vi "Serial.vi"(8 "error in (no error)":errorcluster, 9 "Clear Log":bool, 10 "write buffer":string="UA[3]\r\n", 11 "VISA resource name":refnum<visa-resource-name>="COM6") -> (0 "error out":errorcluster, 2 "read buffer":string, 3 "status":bool)   [LabVIEW 2017]
uses:
  <vilib>/Instr/_visa.llb/VISA Configure Serial Port (Instr).vi
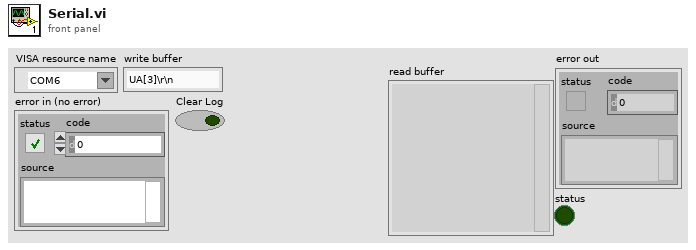
[diagram p1: front panel]
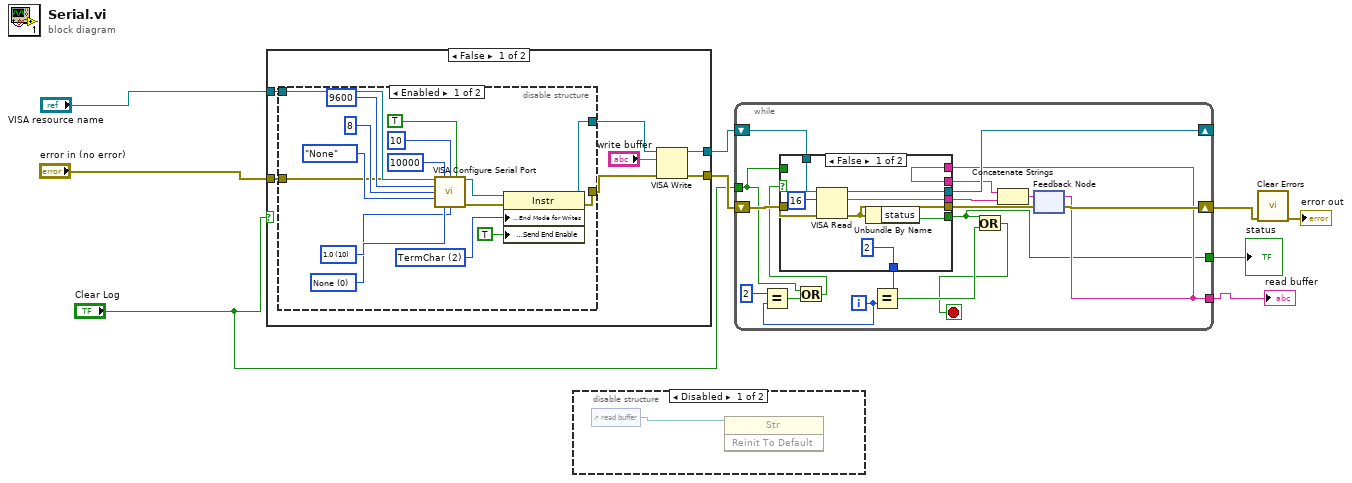
[diagram p0: block diagram]
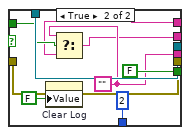
[diagram p5: hidden frame]
diagram:
  n1 = case shown="False" "Clear Log" {
    tunnel: "VISA resource name" -> [w16 w36]
    tunnel: "error in (no error)" -> [w15 w35]
    tunnel: [w12 w36] -> w4
    tunnel: [w11 w35] -> w3
    frame False {
      n2 = disable-structure shown="Enabled" {
        disable-tunnel: w16 -> [w32 w34]
        disable-tunnel: w15 -> [w26 w33]
        disable-tunnel: [w21 w34] -> w13
        disable-tunnel: [w20 w33] -> w14
        frame Enabled {
          w18 = u16 2 items=["None", "LastBit", "TermChar", "Break"] ("Serial Settings:Serial End Mode for Writes")
          w24 = u16 0 items=["None", "XON/XOFF", "RTS/CTS", "XON/XOFF & RTS/CTS", "DTR/DSR", "XON/XOFF & DTR/DSR"] ("flow control (0:none)")
          w25 = u16 10 items=["1.0"=10, "1.5"=15, "2.0"=20] ("stop bits (10: 1 bit)")
          n3 = call-poly "VISA Configure Serial Port"("VISA resource name"=w32, "timeout (10sec)"=u32 10000, "termination char\n(0xA = '\\n' = LF)"=u8 10 ("termination char\n(0xA = '\\n' = LF)"), "Enable Termination\nChar (T)"=TRUE ("Enable Termination\nChar (T)"), "baud rate (9600)"=u32 9600, "data bits (8)"=u16 8, "parity (0:none)"=enum16{"None", "Odd", "Even", "Mark", "Space"}."None", "error in (no error)"=w26, "stop bits (10: 1 bit)"=w25, "flow control (0:none)"=w24) -> ("VISA resource name out"=w22:refnum<visa-resource-name>, "error out"=w23:errorcluster)  [unwired: 4 in]
          n4 = property class="Instr"(reference=w22, error in=w23, "Serial Settings:End Mode for Writes"=w18, "Message Based Settings:Send End Enable"=TRUE) -> (reference out=w21:refnum<visa-resource-name>, error out=w20:errorcluster)
        }
        frame Disabled {
        }
      }
      n5 = VISA Write(VISA resource name=w13, write buffer="write buffer", error in (no error)=w14) -> (VISA resource name out=w12:refnum<visa-resource-name>, error out=w11:errorcluster)  [unwired: 1 out]
    }
    frame True {
    }
  }
  n6 = disable-structure shown="Disabled" {
    frame Disabled {
      n7 = control-ref of="read buffer"() -> (w37:refnum<vi>)
      n8 = invoke class="Str" method="Reinit To Default"(reference=w37) -> ()  [unwired: 2 in, 3 out]
    }
    frame Enabled {
    }
  }
  n9 = while {
    shift-right: [w54] -> _
    shift-left: w4 -> [w49]
    shift-right: [w52] -> w8
    shift-left: w3 -> [w48]
    tunnel: [w46] -> w7
    tunnel: "Clear Log" -> [w39]
    tunnel: [w38] -> w1
    i -> [w43]
    stop <- w50 stop-if-true
    n10 = Equal?(x=2, y=w43) -> (x = y?=w41:bool)
    n11 = Or(x=w39, y=w41) -> (x .or. y?=w40:bool)
    n12 = feedback #1() -> (w46:string)  [unwired: 1 in]
    n13 = case shown="False" w40 {
      tunnel: [w63 w72] -> w54
      tunnel: [w62 w66] -> w53
      tunnel: [w60 w71] -> w52
      tunnel: [w59 FALSE ("status")] -> w38
      tunnel: w49 -> [w58 w72]
      tunnel: w48 -> [w57 w71]
      tunnel: w46 -> [w56 w65]
      tunnel: [w56 w64] -> w45
      tunnel: [2 ("x") 2 ("x")] -> w44
      tunnel: w39 -> [_ w67]
      frame False {
        n14 = VISA Read(VISA resource name=w58, byte count=u32 16, error in (no error)=w57) -> (VISA resource name out=w63:refnum<visa-resource-name>, read buffer=w62:string, error out=w60:errorcluster)  [unwired: 1 out]
        n15 = Unbundle By Name(w60) -> ("status"=w59:bool)
      }
      frame True {
        w66 = ""
        n16 = property on="Clear Log" class="Bool (strict)"("Value"=FALSE ("Clear Log")) -> ()  [unwired: 2 in, 2 out]
        n17 = Select(t=w66, s=w67, f=w65) -> (s? t:f=w64:string)
      }
    }
    n18 = Equal?(x=w44, y=w43) -> (x = y?=w51:bool)
    n19 = Or(x=w38, y=w51) -> (x .or. y?=w50:bool)
    n20 = Concatenate Strings(w45, w53) -> (w47:string)
    n21 = feedback-in #1(w47) -> ()
  }
  "read buffer" <- w7
  "status" <- w1
  n22 = call <vilib>:"Clear Errors.vi"("error in (no error)"=w8) -> ("error out"=→"error out":errorcluster)  [unwired: 5 in, 1 out]
